vi "Interface_Asset_Read Process Name.vi"(11 "EnergyStorage in":refnum<class "EnergyStorage.lvclass">) -> (2 "Process Name":string, 3 "EnergyStorage out":refnum<class "EnergyStorage.lvclass">)   [LabVIEW 2015, in "EnergyStorage.lvclass"]
uses:
  EnergyStorage.lvclass
  EnergyStorage.lvclass/EnergyStorage.ctl
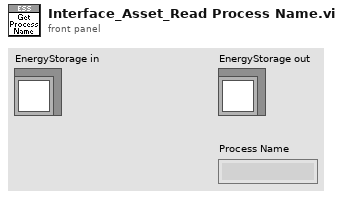
[diagram p1: front panel]
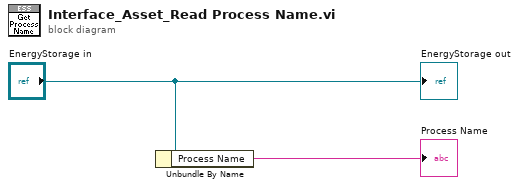
[diagram p0: block diagram]
diagram:
  n1 = Unbundle By Name("EnergyStorage in") -> ("Process Name"=→"Process Name":string)
  "EnergyStorage out" <- "EnergyStorage in"
